vi "DeCoF boolean set.vi"(4 "error in":errorcluster, 5 "value":bool, 6 "param-name":string, 7 "Conncection ID in":T1) -> (0 "error out":errorcluster, 3 "Conncection ID out":T1)   [LabVIEW 2013]
uses:
  DeCoF connection.ctl
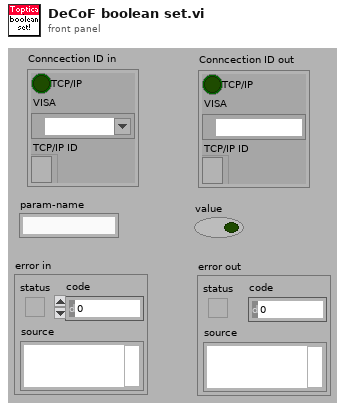
[diagram p1: front panel]
types:
  T1 = typedef "DeCoF connection.ctl" = cluster{"TCP/IP":bool, "VISA":refnum<visa-resource-name>, "TCP/IP ID":refnum<k5>}
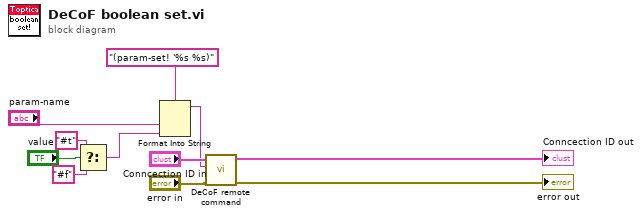
[diagram p0: block diagram]
diagram:
  n1 = Select(t="#t", s="value", f="#f") -> (s? t:f=w1:string)
  n2 = Format Into String(format string="(param-set! '%s %s)", "param-name", w1) -> (resulting string=w6:string)  [unwired: 2 in, 1 out]
  n3 = call "DeCoF remote command.vi"("error in (no error)"="error in", "command"=w6, "Conncection ID in"="Conncection ID in") -> ("error out"=→"error out":errorcluster, "Conncection ID out"=→"Conncection ID out":T1)  [unwired: 2 in, 3 out]
